vi "LCR_Logfile.vi"(4 "Input":T1, 6 "Time Stamp":timestamp format="%<%x %.3X>T", 8 "error in":errorcluster, 9 "Data_In":T2={"Value"=0.0, "GUI Data Cluster"={"SBR"=0}, "Timing"={"Last Operation"=0.0, "Stop @ T"=FALSE, "Delta T Log"=FALSE, "End T"=0.0, "Delta T"=0.0, "Last Temp"=0.0}, "Measurements"=[], "Hardware"={"VNA TCP Port"=5025, "Global T VAR"="", "Global B VAR"=""}} {"GUI Data Cluster"."SBR" format="%08b"}, 10 "Config_In":T4={"General"={"Config.ini"=path "", "Default Logging Path"=path ""}, "Hardware"={"Measure Rate (1/s)"=0, "HP DMM VISA"="", "LS 335 VISA"="", "HP DM"={"Range"=enum."Autorange", "Autozero"=FALSE, "Display"=enum."3 1/2 Digit", "Blank LCD"=FALSE}}, "Operation"={"Operation Mode"=enum."Idle-Off", "Status"="", "NewLog?"=FALSE, "OvenWarn"=FALSE}}) -> (0 "error out":errorcluster, 1 "Data_Out":T2={"Value"=0.0, "GUI Data Cluster"={"SBR"=0}, "Timing"={"Last Operation"=0.0, "Stop @ T"=FALSE, "Delta T Log"=FALSE, "End T"=0.0, "Delta T"=0.0, "Last Temp"=0.0}, "Measurements"=[], "Hardware"={"VNA TCP Port"=5025, "Global T VAR"="", "Global B VAR"=""}} {"GUI Data Cluster"."SBR" format="%08b"}, 2 "Config_Out":T4={"General"={"Config.ini"=path "", "Default Logging Path"=path ""}, "Hardware"={"Measure Rate (1/s)"=0, "HP DMM VISA"="", "LS 335 VISA"="", "HP DM"={"Range"=enum."Autorange", "Autozero"=FALSE, "Display"=enum."3 1/2 Digit", "Blank LCD"=FALSE}}, "Operation"={"Operation Mode"=enum."Idle-Off", "Status"="", "NewLog?"=FALSE, "OvenWarn"=FALSE}}, 3 "File Failure":bool)   [LabVIEW 2021]
uses:
  Mode_Enum.ctl
  Config_Cluster.ctl
  Measurement_Cluster.ctl
  Data_Cluster.ctl
panel:
  in  "Status Ref":refnum<vi>
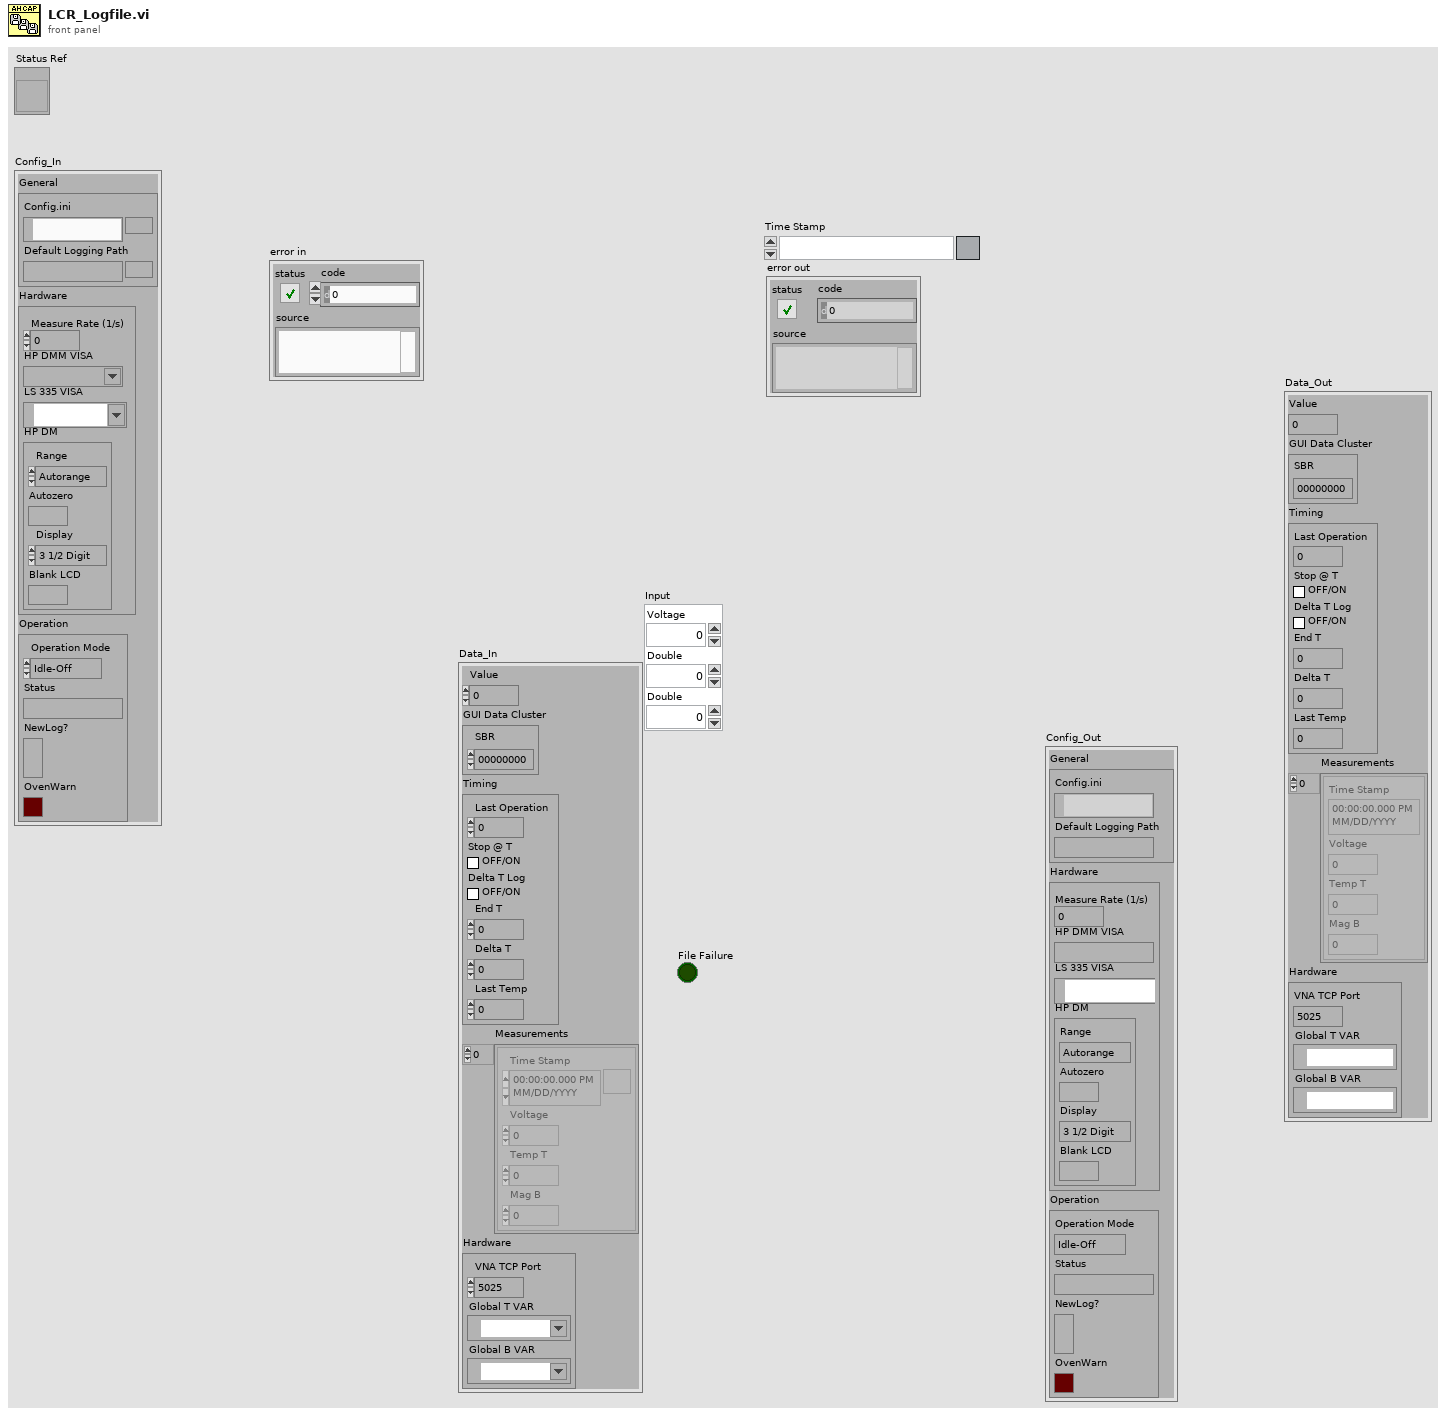
[diagram p1: front panel]
types:
  T1 = cluster{"Voltage":dbl, "Double":dbl, "Double":dbl}
  T2 = typedef "Data_Cluster.ctl" = cluster{"Value":dbl, "GUI Data Cluster":cluster{"SBR":u16}, "Timing":cluster{"Last Operation":dbl, "Stop @ T":bool, "Delta T Log":bool, "End T":dbl, "Delta T":dbl, "Last Temp":dbl}, "Measurements":T3[], "Hardware":cluster{"VNA TCP Port":i32, "Global T VAR":refnum<k21>, "Global B VAR":refnum<k21>}}
  T3 = typedef "Measurement_Cluster.ctl" = cluster{"Time Stamp":timestamp, "Voltage":dbl, "Temp T":dbl, "Mag B":dbl}
  T4 = typedef "Config_Cluster.ctl" = cluster{"General":cluster{"Config.ini":path, "Default Logging Path":path}, "Hardware":cluster{"Measure Rate (1/s)":i32, "HP DMM VISA":refnum<visa-resource-name>, "LS 335 VISA":refnum<visa-resource-name>, "HP DM":cluster{"Range":enum16{"Autorange", "30mV", "300mV", "3V", "30V"}, "Autozero":bool, "Display":enum16{"3 1/2 Digit", "4 1/2 Digit", "5 1/2 Digit"}, "Blank LCD":bool}}, "Operation":cluster{"Operation Mode":T5, "Status":string, "NewLog?":bool, "OvenWarn":bool}}
  T5 = typedef "Mode_Enum.ctl" = enum16{"OvenNRDY", "Logging", "Idle-Off", "Idle"}
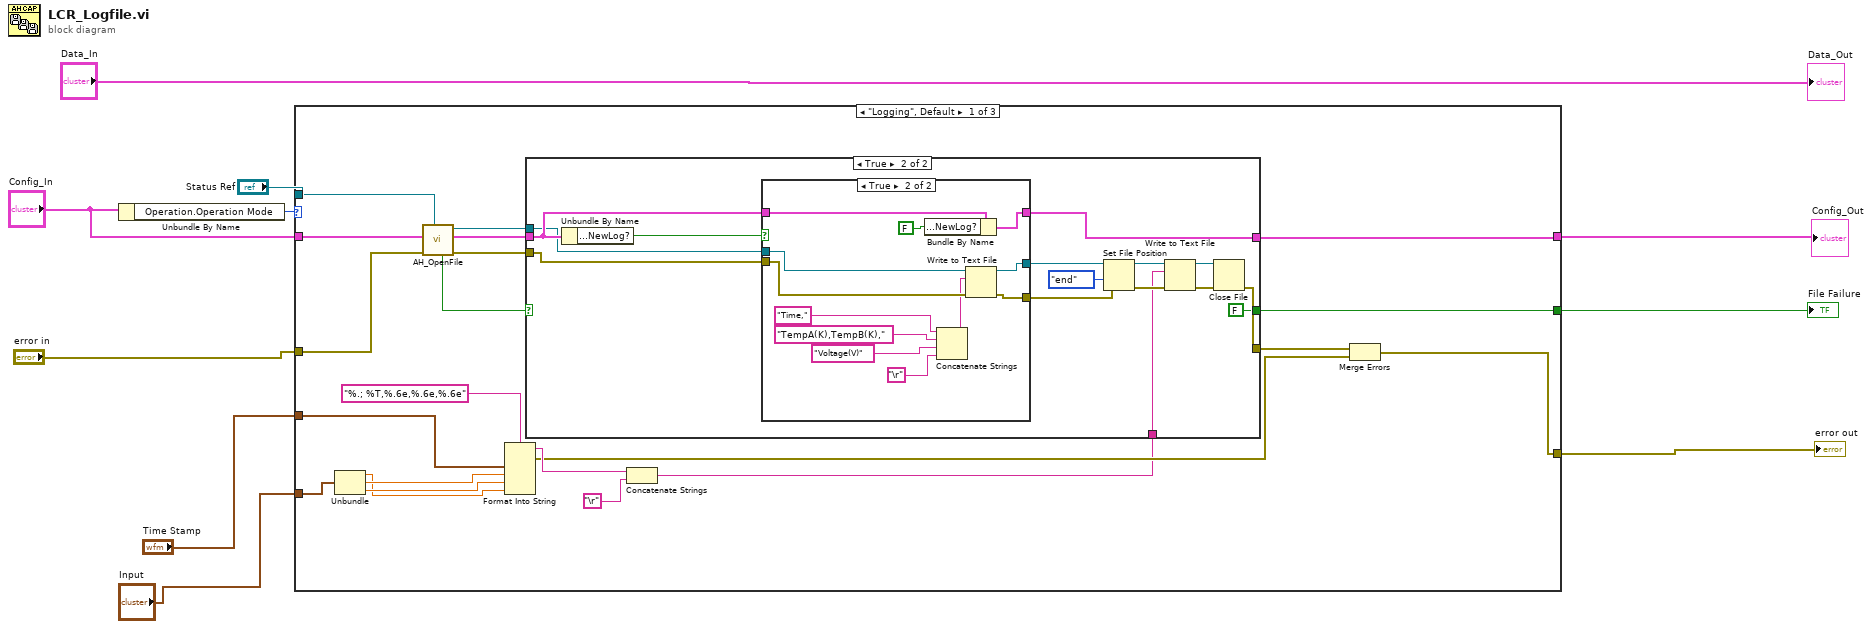
[diagram p0: block diagram]
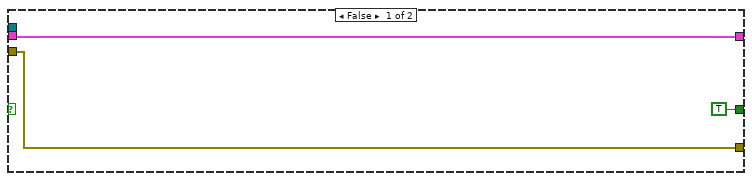
[diagram p2: hidden frame]
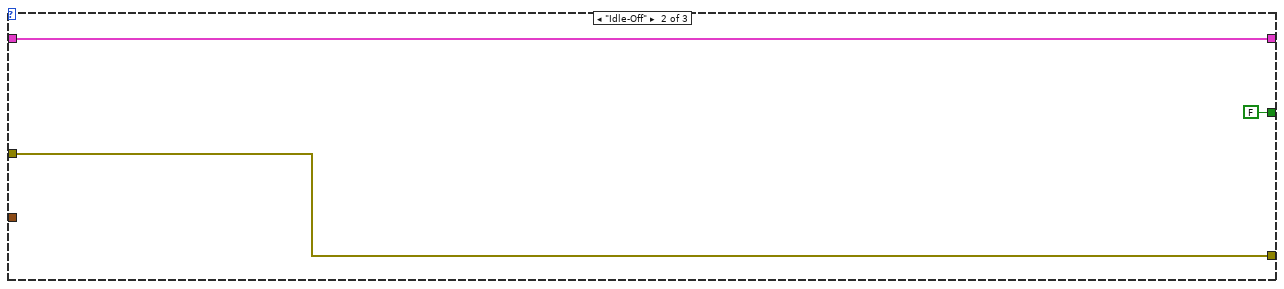
[diagram p4: hidden frame]
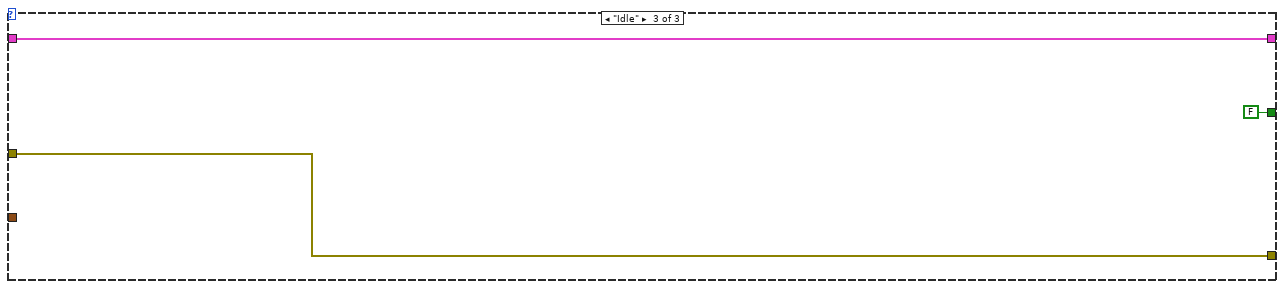
[diagram p5: hidden frame]
diagram:
  n1 = Unbundle By Name("Config_In") -> ("Operation.Operation Mode"=w6:T5)
  n2 = case shown="\"Logging\", Default" w6 {
    tunnel: "error in" -> [w24 w67 w70]
    tunnel: "Time Stamp" -> [w30 _ _]
    tunnel: [w16 w67 w70] -> w9
    tunnel: "Input" -> [w29 _ _]
    tunnel: "Config_In" -> [w26 w66 w69]
    tunnel: "Status Ref" -> [w25 _ _]
    tunnel: [w15 w66 w69] -> w3
    tunnel: [w14 FALSE FALSE] -> w2
    frame "Logging", Default {
      n3 = Unbundle(w29) -> ("Voltage"=w11:dbl, "Double"=w13:dbl, "Double"=w12:dbl)
      n4 = call "AH_OpenFile.vi"("Status Ref"=w25, "error in"=w24, "Config_Cluster"=w26) -> ("error out"=w20:errorcluster, "Config_Cluster Out"=w21:T4, "refnum out"=w22:refnum<file>, "FileOpen?"=w23:bool)  [unwired: 5 in]
      n5 = Format Into String(format string="%.; %T,%.6e,%.6e,%.6e", w30, w13, w12, w11) -> (resulting string=w28:string, error out=w19:errorcluster)  [unwired: 2 in]
      n6 = Concatenate Strings(w28, "\r") -> (w18:string)
      n7 = case shown="True" w23 {
        tunnel: w22 -> [_ w39]
        tunnel: w21 -> [w33 w41]
        tunnel: w20 -> [w34 w38]
        tunnel: w18 -> [_ w43]
        tunnel: [w34 w42] -> w17
        tunnel: [w33 w40] -> w15
        tunnel: [TRUE FALSE] -> w14
        frame False {
        }
        frame True {
          n8 = Unbundle By Name(w41) -> ("Operation.NewLog?"=w49:bool)
          n9 = case shown="True" w49 {
            tunnel: w41 -> [w52 w64]
            tunnel: [w52 w63] -> w40
            tunnel: w39 -> [w51 w59]
            tunnel: w38 -> [w50 w58]
            tunnel: [w51 w61] -> w37
            tunnel: [w50 w60] -> w36
            frame False {
            }
            frame True {
              n10 = Bundle By Name(cluster=w64, "Operation.NewLog?"=FALSE) -> (w63:T4)
              n11 = Concatenate Strings("Time,", "TempA(K),TempB(K),", "Voltage(V)" ("string"), "\r") -> (w56:string)
              n12 = Write to Text File(file (use dialog)=w59, text=w56, error in=w58) -> (refnum out=w61:refnum<file>, error out=w60:errorcluster)  [unwired: 1 in, 1 out]
            }
          }
          n13 = Set File Position(refnum=w37, from (0:start)=enum16{"start", "end", "current"}."end", error in=w36) -> (refnum out=w47:refnum<file>, error out=w48:errorcluster)  [unwired: 1 in]
          n14 = Write to Text File(file (use dialog)=w47, text=w43, error in=w48) -> (refnum out=w46:refnum<file>, error out=w45:errorcluster)  [unwired: 1 in, 1 out]
          n15 = Close File(refnum=w46, error in=w45) -> (error out=w42:errorcluster)  [unwired: 1 out]
        }
      }
      n16 = Merge Errors(w17, w19) -> (w16:errorcluster)
    }
    frame "Idle-Off" {
    }
    frame "Idle" {
    }
  }
  "error out" <- w9
  "Config_Out" <- w3
  "File Failure" <- w2
  "Data_Out" <- "Data_In"
